vi "Calculate Nominal Resistance.vi"(0 "Digit":T1, 2 "Digit 2":T1, 3 "Digit 3":T1, 4 "Numero de bandas":T2=5 min=3 max=6 step=1, 5 "Multiplier":T3) -> (7 "Nominal":dbl)   [LabVIEW 2018]
uses:
  Digit--control.ctl
  Multiplier--control.ctl
  Number of bands.ctl
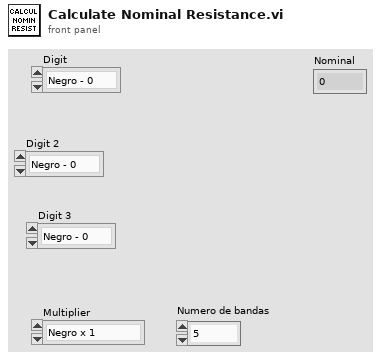
[diagram p1: front panel]
types:
  T1 = typedef "Digit--control.ctl" = enum16{"Negro - 0", "Marron - 1", "Rojo - 2", "Naranja - 3", "Amarillo - 4", "Verde - 5", "Azul - 6", "Violeta - 7", "Gris - 8", "Blanco - 9"}
  T2 = typedef "Number of bands.ctl" = u8
  T3 = typedef "Multiplier--control.ctl" = enum16{"Negro x 1", "Marron x 10", "Rojo x 100", "Naranja x 1K", "Amarillo x 10K", "Verde x 100K", " Azul x 1M", "Violeta x 10M ", "Oro x 0.1", "Plata x 0.01"}
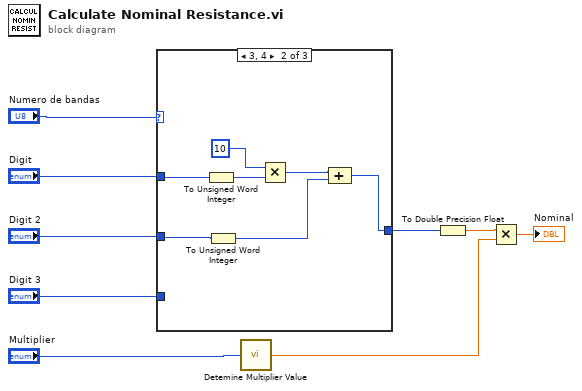
[diagram p0: block diagram]
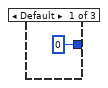
[diagram p2: hidden frame]
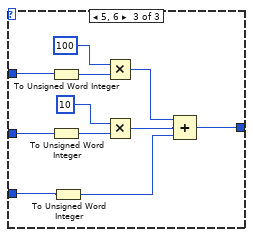
[diagram p3: hidden frame]
diagram:
  n1 = case shown="3, 4" "Numero de bandas" {
    tunnel: "Digit" -> [_ w13 w26]
    tunnel: "Digit 2" -> [_ w12 w23]
    tunnel: "Digit 3" -> [_ _ w22]
    tunnel: [u16 0 w11 w18] -> w4
    frame Default {
    }
    frame 3, 4 {
      n2 = To Unsigned Word Integer(number=w13) -> (unsigned 16bit integer=w16:u16)
      n3 = To Unsigned Word Integer(number=w12) -> (unsigned 16bit integer=w14:u16)
      n4 = Multiply(x=u16 10, y=w16) -> (x*y=w15:u16)
      n5 = Compound Arithmetic op=ADD(w15, w14) -> (w11:u16)
    }
    frame 5, 6 {
      n6 = To Unsigned Word Integer(number=w26) -> (unsigned 16bit integer=w28:u16)
      n7 = To Unsigned Word Integer(number=w23) -> (unsigned 16bit integer=w24:u16)
      n8 = To Unsigned Word Integer(number=w22) -> (unsigned 16bit integer=w19:u16)
      n9 = Multiply(x=u16 100, y=w28) -> (x*y=w21:u16)
      n10 = Multiply(x=u16 10, y=w24) -> (x*y=w20:u16)
      n11 = Compound Arithmetic op=ADD(w21, w20, w19) -> (w18:u16)
    }
  }
  n12 = call "Detemine Multiplier Value.vi"("Multiplier"="Multiplier") -> ("Numeric"=w2:dbl)  [unwired: 4 in]
  n13 = To Double Precision Float(number=w4) -> (double precision float=w3:dbl)
  n14 = Multiply(x=w3, y=w2) -> (x*y=→"Nominal":dbl)
